vi "SendNetworkVariant.vi"(0 "reference in":refnum<class "MessageInterface.lvclass">, 1 "receiver process":string, 2 "receiver host":string, 3 "receiver port (0)":u16, 5 "name":string, 7 "data":variant, 9 "timeout (25000 ms)":i32=25000, 11 "error in (no error)":errorcluster) -> (4 "reference out":refnum<class "MessageInterface.lvclass">, 10 "timed out?":bool, 15 "error out":errorcluster)   [LabVIEW 2019, in "MessageInterface.lvclass"]
uses:
  MessageInterface.lvclass
  <vilib>/addons/_JKI.lib/Serialization/JSON/Library/Flatten To JSON String.vi
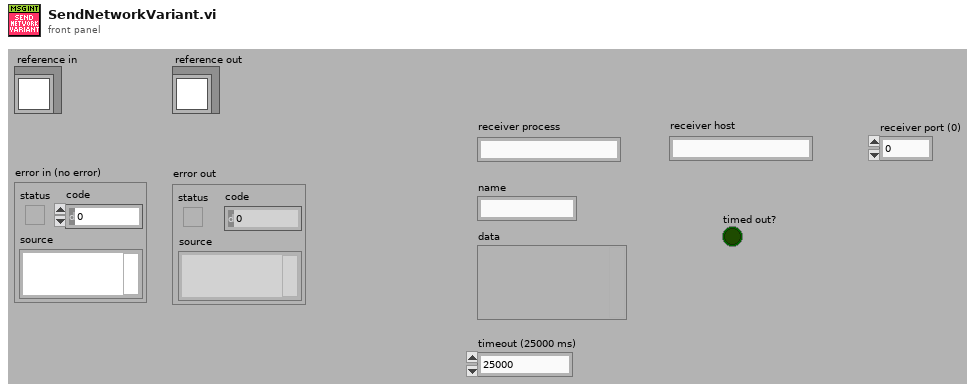
[diagram p1: front panel]
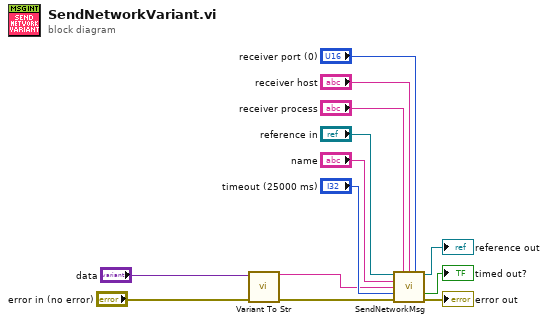
[diagram p0: block diagram]
diagram:
  n1 = call "Variant To Str.vi"("data"="data", "error in (no error)"="error in (no error)") -> ("JSON String"=w3:string, "error out"=w7:errorcluster)  [unwired: 12 in]
  n2 = call-dynamic "SendNetworkMsg.vi"("reference in"="reference in", "receiver process"="receiver process", "receiver host"="receiver host", "receiver port (0)"="receiver port (0)", "name"="name", "value"=w3, "timeout (25000 ms)"="timeout (25000 ms)", "error in (no error)"=w7) -> ("reference out"=→"reference out":refnum<class "MessageInterface.lvclass">, "timed out?"=→"timed out?":bool, "error out"=→"error out":errorcluster)  [unwired: 5 in]
